vi "Stop Core.vi"(10 "最终错误代码":i32, 11 "冷却器的控制器输入":refnum<class "Cooler Controller.lvclass">) -> (3 "冷却器的控制器输出":refnum<class "Cooler Controller.lvclass">)   [LabVIEW 2013, in "Cooler Controller.lvlib" / "Cooler Controller.lvclass"]
doc: "对于操作者运行过程中创建的所有并行进程，在重写Stop Core.vi的VI中应调用必要代码使其停止运行。需要停止的进程包括该操作本身创建的层层嵌套的操作者，以及所有其他异步运行的VI，比如时间延迟消息。需要停止的进程可能还包括Actor Core中的所有并行循环。（另一种方法，是在Actor Core程序框图上，在“调用父节点”结束时触发一个局部信号来停止这些进程。）\n\n<b>最终错误代码</b>输入表示操作者退出时设定的错误。0表示无错误。该错误代码可用于区分“正常停止”和“紧急停止”，从而向其他操作者发送信号。一般用非零值表示“紧急停止”，当然对于某个特定的操作者也可采用其他的表示方法。请注意，1608是个特殊的错误代码，表示当前操作者本身被“紧急停止”，如出现该错误，只能直接传递该代码。"
uses:
  Cooler Controller.lvclass
  <vilib>/ActorFramework/Actor/Actor.lvclass
  Cooler Controller.lvclass/Cooler Controller.ctl
  <vilib>/ActorFramework/Stop Msg/Stop Msg.lvclass/Stop Msg.ctl
  <vilib>/ActorFramework/Message Enqueuer/Message Enqueuer.lvclass/Message Enqueuer.ctl
  <vilib>/ActorFramework/Message Enqueuer/Enqueue Critical.vi
  <vilib>/ActorFramework/Message Priority Queue/Priority Enqueue.vi
  <vilib>/ActorFramework/Stop Msg/Stop Msg.lvclass
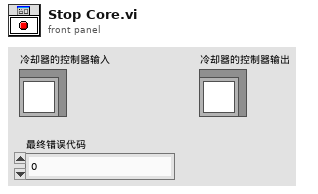
[diagram p1: front panel]
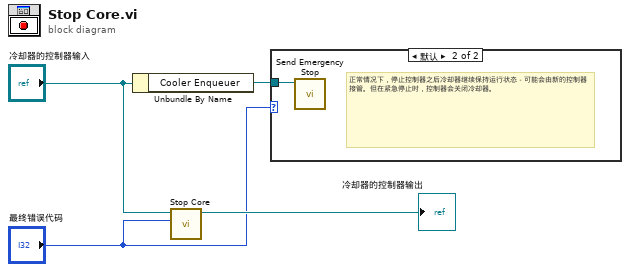
[diagram p0: block diagram]
diagram:
  n1 = Unbundle By Name("冷却器的控制器输入") -> ("Cooler Enqueuer"=w3:refnum<class "Message Enqueuer.lvclass">)
  n2 = call-parent "Stop Core.vi"("final error code"="最终错误代码", "Actor in"="冷却器的控制器输入") -> ("Actor out"=→"冷却器的控制器输出":refnum<class "Cooler Controller.lvclass">)  [unwired: 9 in]
  n3 = case shown="默认" "最终错误代码" {
    tunnel: w3 -> [_ w5]
    frame 0 {
      # "正常停止时冷却器保持运行状态。"
    }
    frame Default {
      # "正常情况下，停止控制器之后冷却器继续保持运行状态－可能会由新的控制器接管。但在紧急停止时，控制器会关闭冷却器。"
      n4 = call <vilib>:"Send Emergency Stop.vi"("Message Enqueuer"=w5) -> ()  [unwired: 10 in, 1 out]
    }
  }
